vi "Send message.vi"(8 "error in (no error)":errorcluster, 10 "message":T1, 11 "Messenger in":refnum<class "Messenger.lvclass">) -> (0 "error out":errorcluster, 3 "Messenger out":refnum<class "Messenger.lvclass">)   [LabVIEW 2018, in "Messenger.lvclass"]
uses:
  Messenger.lvclass
  Message Queue/Message Cluster.ctl
  Messenger.lvclass/Messenger.ctl
  Message Queue/Message Queue.lvlib
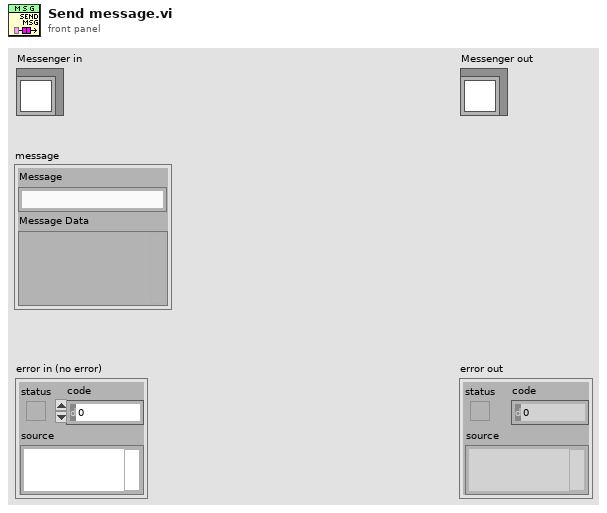
[diagram p1: front panel]
types:
  T1 = typedef "Message Queue.lvlib/Message Cluster.ctl" = cluster{"Message":string, "Message Data":variant}
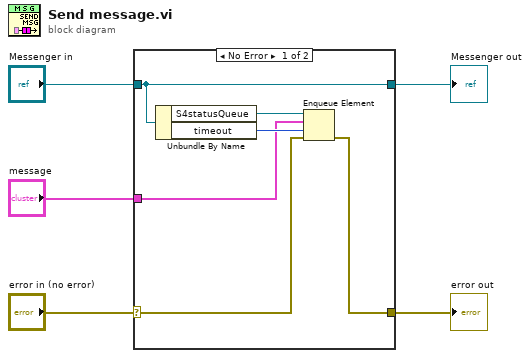
[diagram p0: block diagram]
diagram:
  n1 = case shown="No Error" "error in (no error)" {
    selector: "error in (no error)" -> [w9 w12]
    tunnel: [w7 w12] -> w4
    tunnel: [w11 w13] -> w2
    tunnel: "Messenger in" -> [w11 w13]
    tunnel: "message" -> [w6 _]
    frame No Error {
      n2 = Unbundle By Name(w11) -> ("S4statusQueue"=w10:refnum<queue>, "timeout"=w8:i32)
      n3 = Enqueue Element(queue=w10, element=w6, timeout in ms (-1)=w8, error in (no error)=w9) -> (error out=w7:errorcluster)  [unwired: 2 out]
    }
    frame Error {
    }
  }
  "error out" <- w4
  "Messenger out" <- w2
